vi "Intellirupter_main_WVM.vi"() -> ()   [LabVIEW 2016]
uses:
  <vilib>/Platform/TimedLoop/XDataNode/timing_clust.ctl
  <vilib>/Platform/TimedLoop/XDataNode/nitl_modes.ctl
  <vilib>/Platform/TimedLoop/XDataNode/wakeup.ctl
  <vilib>/FPGAPlugInAG/cRIO-9039 (Sync)/niLvFpga_Open_cRIO-9039 (Sync).vi
  <vilib>/rvi/interface/common/dynamic/niFpgaDynamicAddResources.vi
  <vilib>/Utility/error.llb/Error Cluster From Error Code.vi
  <vilib>/rvi/errors/niLvFpgaAdjustHostInterfaceError.vi
  <vilib>/FPGAPlugInAG/Dynamic/niLvFpga_Close_Dynamic.vi
  <vilib>/rvi/interface/nirviOpenFPGA/nirviOpenFPGA.xnode
  FPGA Bitfiles/IntelliRupter_calibrated.lvbitx
  <vilib>/rvi/interface/nirviReadWriteControl/nirviReadWriteControl.xnode
  <vilib>/Platform/TimedLoop/XDataNode/XDataNode.xnode
  <vilib>/rvi/interface/nirviCloseFPGA/nirviCloseFPGA.xnode
  <vilib>/rvi/interface/Simulation/niFpgaSimulationCallBeginRW.vi
  NiFpgaLv.dll
  <vilib>/Platform/TimedLoop/XDataNode/XDNodeRunTimeDep.lvlib
panel:
  out "basic calc interval":u16=2028
  out "half cycle (samples)":i32=96
  out "Waveform Chart 2":dbl(graph)=58.831625507750715
  in  "I offset R2":dbl=-0.005
  in  "I offset R7":dbl=-0.04
  in  "I offset R3":dbl=-0.12
  out "R8 Transfer":bool
  out "R7 Transfer":bool
  out "R5 Transfer":bool
  out "R4 Transfer":bool
  out "R2 Transfer":bool
  in  "I offset R8":dbl=0.091
  in  "I offset R4":dbl
  in  "I offset R6":dbl=0.092
  in  "I offset R5":dbl=0.035
  in  "I offset R1":dbl=-0.14
  in  "R8 Blocking in":bool
  in  "R7 Blocking in":bool
  in  "R6 Blocking in":bool
  in  "R5 Blocking in":bool
  in  "R4 Blocking in":bool
  in  "R3 Blocking in":bool
  in  "R2 Blocking in":bool
  in  "R1 Blocking in":bool
  out "R1 Blocking out":bool[](array[boolean])
  out "R2 Blocking out":bool[](array[boolean])
  out "R3 Blocking out":bool[](array[boolean])
  out "R4 Blocking out":bool[](array[boolean])
  out "R5 Blocking out":bool[](array[boolean])
  out "R6 Blocking out":bool[](array[boolean])
  out "R8 Blocking out":bool[](array[boolean])
  out "R7 Blocking out":bool[](array[boolean])
  out "Relay7 Reclose":bool=TRUE
  out "Relay7 Trip":bool
  out "Relay8 Reclose":bool=TRUE
  out "Relay8 Trip":bool
  out "Relay6 Reclose":bool=TRUE
  out "Relay6 Trip":bool
  out "Relay5 Reclose":bool=TRUE
  out "Relay5 Trip":bool
  out "Relay4 Reclose":bool=TRUE
  out "Relay4 Trip":bool
  out "Relay3 Reclose":bool=TRUE
  out "Relay3 Trip":bool
  out "Relay2 Reclose":bool=TRUE
  out "Relay2 Trip":bool
  out "Relay1 Reclose":bool=TRUE
  out "Relay1 Trip":bool
  in  "Manual Relay Control":bool
  in  "Reset Relay":bool
  out "Loop time":u32=60
  in  "Recloser Settings":T1={"Magnitude Minimum"=0.1, "Magnitude difference level"=0.1, "Frequency difference level"=0.5, "Phase difference level"=10.0}
  out "MGCC_to_relay":bool[](array[boolean])=[TRUE, TRUE, FALSE, TRUE, TRUE, TRUE, TRUE, TRUE]
  in  "Count(ticks)":u32=10000
  in  "RMS minimum\nvalues":cluster{"VRMS values":dbl, "IRMS values":dbl}={"VRMS values"=0.1, "IRMS values"=0.1}
  out "error out":errorcluster
  out "Relay_toMGCC":bool[](array[boolean])=[TRUE, TRUE, FALSE, TRUE, TRUE, TRUE, TRUE, TRUE]
  in  "Reclose Relay8?":bool=TRUE
  out "R8 Data for\ncommunication":dbl[](array[numeric])=[1.0, 0.9862955093401103, 0.9867214322763603, 58.77451863285861, 58.803693074154864, -0.7941289762119178, 0.09008148312568665, 0.0005073295324109495, 0.0, 0.0]
  in  "Reclose Relay7?":bool=TRUE
  out "R7 Data for\ncommunication":dbl[](array[numeric])=[1.0, 0.9866141364364692, 0.9877614986081782, 58.78358722132554, 58.78069274736454, -1.3449540750541662, 0.08266890794038773, 0.0049254209734499454, 0.0, 0.0]
  in  "Reclose Relay6?":bool=TRUE
  out "R6 Data for\ncommunication":dbl[](array[numeric])=[1.0, 0.9875353501134793, 0.9865248048931855, 58.785757996057974, 58.787154979347115, -1.8287701023872671, 0.08318708091974258, 0.007122902199625969, 0.0, 0.0]
  in  "Reclose Relay5?":bool=TRUE
  out "R5 Data for\ncommunication":dbl[](array[numeric])=[1.0, 0.9886971641324518, 0.9869546019014549, 58.82457095733067, 58.82031783160583, -1.940448004694133, 0.2878004312515259, 0.005543795879930258, 0.0, 0.0]
  in  "Reclose Relay4?":bool=TRUE
  out "R4 Data for\ncommunication":dbl[](array[numeric])=[1.0, 0.9905203551104792, 0.9879386593373192, 58.82435803722625, 58.82419110288083, 1.1327042471490738, 0.28807735443115234, 0.028975406661629677, 0.0, 0.0]
  in  "Reclose Relay3?":bool
  out "R3 Data for\ncommunication":dbl[](array[numeric])=[0.0, 0.9908674808017178, 0.002941768314579481, 81.08898160573632, 58.80421372524394, 60.0, -0.0007620751857757568, -9.880386642180383e-06, 0.0, 0.0]
  in  "Reclose Relay2?":bool=TRUE
  out "R2 Data for\ncommunication":dbl[](array[numeric])=[1.0, 0.9909485571563869, 0.9904603427539119, 58.813573202375395, 58.79227178425196, 0.9332438342282595, 0.38369542360305786, 0.024205466732382774, 0.0, -0.021301418123435667]
  out "R1 Data for\ncommunication":dbl[](array[numeric])=[1.0, 0.9931811773356323, 0.9935607508678418, 58.852139713340016, 58.831625507750715, 0.5044340052335675, 0.4828683137893677, 0.0162374097853899, 0.0, -0.020514205589300616]
  in  "Relay8":bool=TRUE
  in  "Relay7":bool=TRUE
  in  "Relay6":bool=TRUE
  in  "Relay5":bool=TRUE
  in  "Relay4":bool=TRUE
  in  "Relay3":bool
  in  "Relay2":bool=TRUE
  in  "Reclose Relay1?":bool=TRUE
  in  "stop":bool
  in  "Relay1":bool=TRUE
  # "status\nmag_left\nmag_right\nfreq_left\nfreq_right\nang_diff\nact_power\nrea_power\n0\n0"
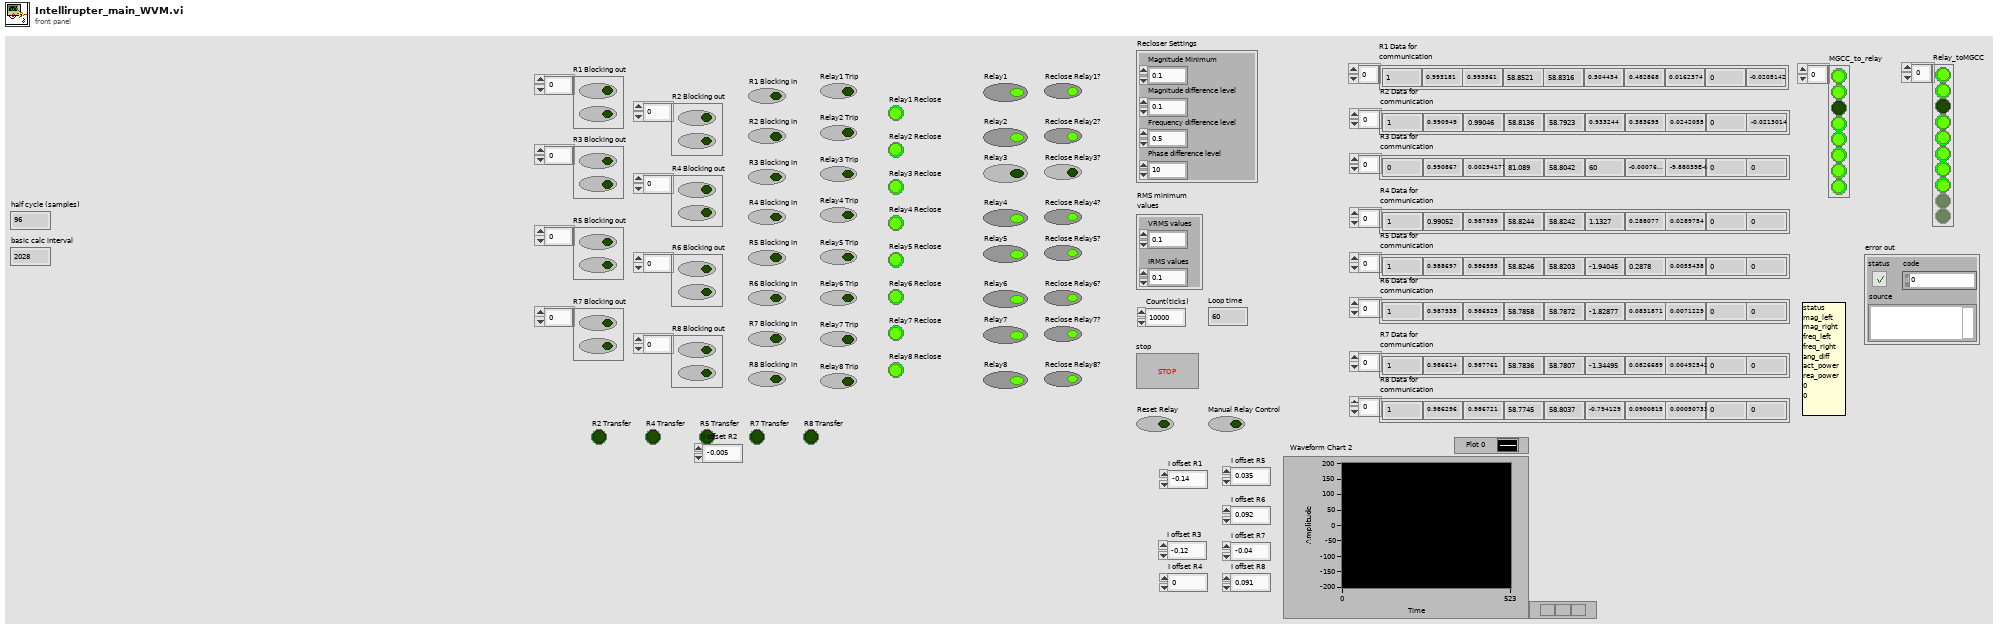
[diagram p1: front panel]
types:
  T1 = cluster{"Magnitude Minimum":dbl, "Magnitude difference level":dbl, "Frequency difference level":dbl, "Phase difference level":dbl}
  T2 = typedef "XDNodeRunTimeDep.lvlib/timing_clust.ctl" = cluster{"Expected End [f-1]":u64, "Actual End [f-1]":u64, "Finished Late? [f-1]":bool, "Expected End [i-1]":u64, "Actual End [i-1]":u64, "Finished Late? [i-1]":bool, "Expected Start [i]":u64, "Actual Start [i]":u64, "Expected Start [f]":u64, "Actual Start [f]":u64, "Source Name":string, "Structure Name":string, "Period":i64, "Deadline":i64, "Offset":i64, "Start":i64, "Priority":i32, "Timeout":i32, "Mode":T3, "Wakeup Reason":T4, "Error":errorcluster, "Source Type":string, "Secondary Source Type":string, "Global End Time":u64, "Global Start Time":u64, "Frame Duration":u64, "Iteration Duration":u64, "Assigned CPU":i32, "I/O Scan Engine Mode":u32}
  T3 = typedef "XDNodeRunTimeDep.lvlib/nitl_modes.ctl" = enum32{"No Change", "Process missed periods, maintain original phase", "Discard missed periods, maintain original phase", "Process missed periods, ignore original phase", "Discard missed periods, ignore original phase"}
  T4 = typedef "XDNodeRunTimeDep.lvlib/wakeup.ctl" = enum32{"Normal", "Aborted", "Asynchronous wakeup", "Timing source error", "Timed loop error", "Timeout"}
  T5 = enum16{"Grid-connected", "BESS only", "PV + BESS"}
  T6 = cluster{"UV Reset level":dbl, "Undervoltage \npick-up level":dbl, "OC Reset level":dbl, "Overcurrent\npick-up level":dbl, "time delay settings":cluster{"Definite operate time [ms]":u32, "Inverse Operating Time [ms]":u32, "reset time [ms]":u32, "operate time compensation [ms]":u32}}
  T7 = cluster{fxp<+/-,53,11>[], fxp<+/-,53,11>[], fxp<+/-,53,11>[], fxp<+/-,53,11>[], fxp<+/-,53,11>[], fxp<+/-,53,11>[], fxp<+/-,53,11>[], fxp<+/-,53,11>[], fxp<+/-,53,11>[]}
  T8 = typedef "NI_EP_Protection_FPGA.lvlib/fpga_Timer Feedback Var.ctl" = cluster{"time elapsed":u32, "start time of trip counting":u32, "start time of reseting":u32}
  T9 = typedef "NI_EP_Protection_FPGA.lvlib/fpga_State.ctl" = enum16{"Idle", "Trip Counting", "Tripped", "Reset Counting"}
  T10 = cluster{"Direction":enum16{"forward", "backward", "N/D"}, "Boolean":bool, "timing values out":T8, "status out":T9, "trip signal out":bool, "State Out":enum16{"Idle", "Wait for Trip", "PulseClosing", "Locked"}, "Pulse Index Out":i32, "start time of reseting":u32}
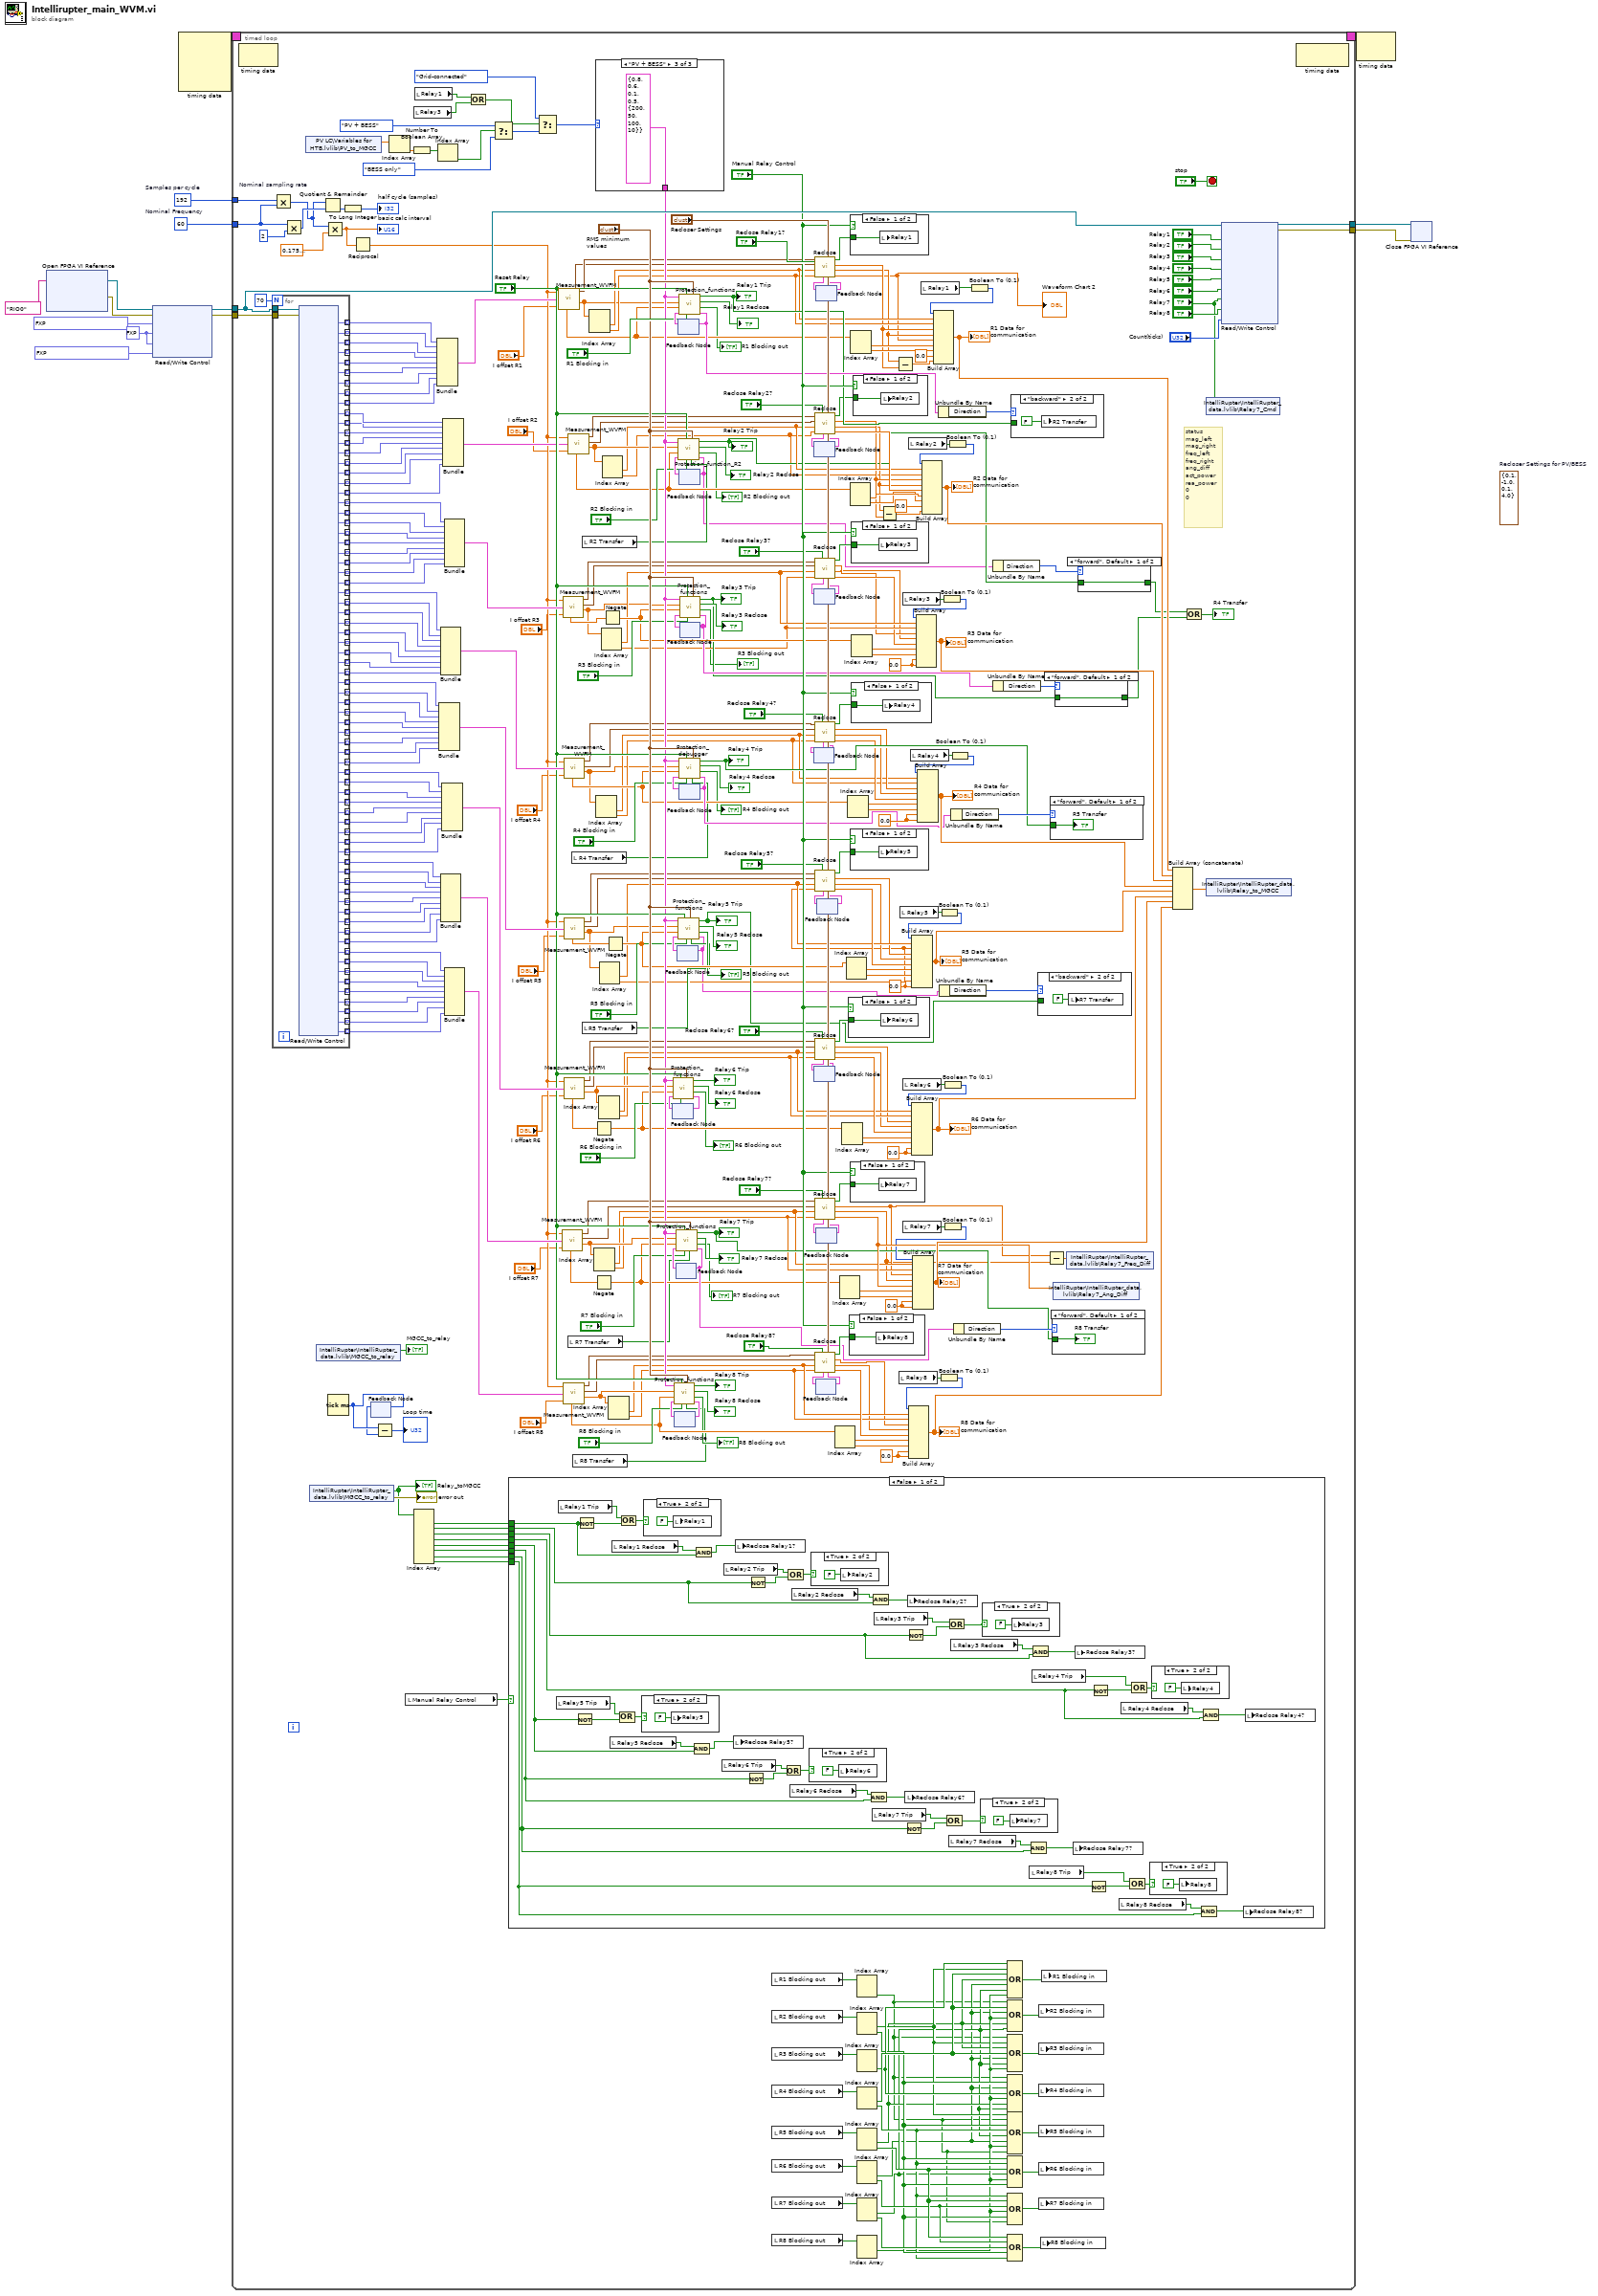
[diagram p0: block diagram]
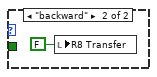
[diagram p2: hidden frame]
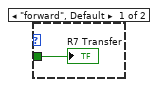
[diagram p3: hidden frame]
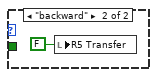
[diagram p4: hidden frame]
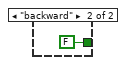
[diagram p5: hidden frame]
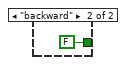
[diagram p6: hidden frame]
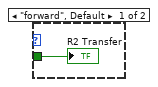
[diagram p7: hidden frame]
diagram:
  w2 = 192  # Samples per cycle
  w1 = 60  # Nominal Frequency
  (unwired) T1 {"Magnitude Minimum"=0.1, "Magnitude difference level"=-1.0, "Frequency difference level"=0.1, "Phase difference level"=4.0}  # Recloser Settings for PV/BESS
  w6 = fxp<+/-,52,10> 0.0 ("I offset")
  n1 = xnode "Open FPGA VI Reference"("resource name"=tag "RIO0") -> ("FPGA VI Reference Out"=w5:refnum<k20>, "error out"=w10:errorcluster)  [unwired: 1 in]
  n2 = xnode "Read/Write Control"("FPGA VI Reference In"=w5, "error in"=w10, "I scale factor"=fxp<+/-,26,5> 0.4850001335144043, "I offset"=w6, "V offset"=w6, "V scale factor"=fxp<+/-,26,5> 0.40000009536743164) -> ("FPGA VI Reference Out"=w11:refnum<k20>, "error out"=w9:errorcluster)
  n3 = node-c288() -> (w4:T2)  [unwired: 4 in]
  n4 = timed-loop {
    tunnel: w11 -> [w407]
    tunnel: [w409] -> w13
    tunnel: [w408] -> w12
    tunnel: w9 -> [w406]
    timing: w4 -> [_]
    timing-out: [_] -> w3
    tunnel: w2 -> [w86]
    tunnel: w1 -> [w85]
    stop <- "stop" stop-if-true
    w243 = 0.0 ("element")
    w244 = 0.0 ("element")
    w256 = 0.0 ("element")
    w127 = 0.0 ("element")
    w268 = 0.0 ("element")
    w269 = 0.0 ("element")
    # "status\nmag_left\nmag_right\nfreq_left\nfreq_right\nang_diff\nact_power\nrea_power\n0\n0"
    n5 = node-c288() -> ()  [unwired: 1 in, 1 out]
    n6 = for {
      N: 70 -> [_]
      tunnel: w407 -> [w484]
      tunnel: w406 -> [w483]
      tunnel: [w482] -> w405 mode=indexing
      tunnel: [w481] -> w404 mode=indexing
      tunnel: [w480] -> w403 mode=indexing
      tunnel: [w479] -> w402 mode=indexing
      tunnel: [w478] -> w401 mode=indexing
      tunnel: [w477] -> w400 mode=indexing
      tunnel: [w476] -> w399 mode=indexing
      tunnel: [w475] -> w398 mode=indexing
      tunnel: [w474] -> w386 mode=indexing
      tunnel: [w473] -> w385 mode=indexing
      tunnel: [w472] -> w384 mode=indexing
      tunnel: [w471] -> w383 mode=indexing
      tunnel: [w470] -> w382 mode=indexing
      tunnel: [w469] -> w381 mode=indexing
      tunnel: [w468] -> w380 mode=indexing
      tunnel: [w467] -> w379 mode=indexing
      tunnel: [w466] -> w378 mode=indexing
      tunnel: [w465] -> w377 mode=indexing
      tunnel: [w464] -> w376 mode=indexing
      tunnel: [w463] -> w375 mode=indexing
      tunnel: [w462] -> w374 mode=indexing
      tunnel: [w461] -> w373 mode=indexing
      tunnel: [w460] -> w372 mode=indexing
      tunnel: [w459] -> w371 mode=indexing
      tunnel: [w458] -> w370 mode=indexing
      tunnel: [w457] -> w369 mode=indexing
      tunnel: [w456] -> w368 mode=indexing
      tunnel: [w455] -> w367 mode=indexing
      tunnel: [w454] -> w366 mode=indexing
      tunnel: [w453] -> w365 mode=indexing
      tunnel: [w452] -> w364 mode=indexing
      tunnel: [w451] -> w363 mode=indexing
      tunnel: [w450] -> w362 mode=indexing
      tunnel: [w449] -> w361 mode=indexing
      tunnel: [w448] -> w360 mode=indexing
      tunnel: [w447] -> w359 mode=indexing
      tunnel: [w446] -> w358 mode=indexing
      tunnel: [w445] -> w357 mode=indexing
      tunnel: [w444] -> w356 mode=indexing
      tunnel: [w443] -> w355 mode=indexing
      tunnel: [w442] -> w354 mode=indexing
      tunnel: [w441] -> w353 mode=indexing
      tunnel: [w440] -> w352 mode=indexing
      tunnel: [w439] -> w351 mode=indexing
      tunnel: [w438] -> w350 mode=indexing
      tunnel: [w437] -> w349 mode=indexing
      tunnel: [w436] -> w348 mode=indexing
      tunnel: [w435] -> w347 mode=indexing
      tunnel: [w434] -> w346 mode=indexing
      tunnel: [w433] -> w345 mode=indexing
      tunnel: [w432] -> w344 mode=indexing
      tunnel: [w431] -> w343 mode=indexing
      tunnel: [w430] -> w342 mode=indexing
      tunnel: [w429] -> w341 mode=indexing
      tunnel: [w428] -> w340 mode=indexing
      tunnel: [w427] -> w339 mode=indexing
      tunnel: [w426] -> w338 mode=indexing
      tunnel: [w425] -> w337 mode=indexing
      tunnel: [w424] -> w336 mode=indexing
      tunnel: [w423] -> w335 mode=indexing
      tunnel: [w422] -> w334 mode=indexing
      tunnel: [w421] -> w333 mode=indexing
      tunnel: [w420] -> w280 mode=indexing
      tunnel: [w419] -> w184 mode=indexing
      tunnel: [w418] -> w183 mode=indexing
      tunnel: [w417] -> w182 mode=indexing
      tunnel: [w416] -> w181 mode=indexing
      tunnel: [w415] -> w180 mode=indexing
      tunnel: [w414] -> w179 mode=indexing
      tunnel: [w413] -> w178 mode=indexing
      tunnel: [w412] -> w177 mode=indexing
      tunnel: [w411] -> w176 mode=indexing
      n7 = xnode "Read/Write Control"("FPGA VI Reference In"=w484, "error in"=w483) -> ("V1L AB"=w420:fxp<+/-,53,11>, "V1L BC"=w482:fxp<+/-,53,11>, "V1L CA"=w481:fxp<+/-,53,11>, "V1R AB"=w480:fxp<+/-,53,11>, "V1R BC"=w479:fxp<+/-,53,11>, "V1R CA"=w478:fxp<+/-,53,11>, "I1 A"=w477:fxp<+/-,53,11>, "I1 B"=w476:fxp<+/-,53,11>, "I1 C"=w475:fxp<+/-,53,11>, "V2L AB"=w419:fxp<+/-,53,11>, "V2L BC"=w418:fxp<+/-,53,11>, "V2L CA"=w417:fxp<+/-,53,11>, "V2R AB"=w416:fxp<+/-,53,11>, "V2R BC"=w415:fxp<+/-,53,11>, "V2R CA"=w414:fxp<+/-,53,11>, "I2 A"=w413:fxp<+/-,53,11>, "I2 B"=w412:fxp<+/-,53,11>, "I2 C"=w411:fxp<+/-,53,11>, "V3L AB"=w474:fxp<+/-,53,11>, "V3L BC"=w473:fxp<+/-,53,11>, "V3L CA"=w472:fxp<+/-,53,11>, "V3R AB"=w471:fxp<+/-,53,11>, "V3R BC"=w470:fxp<+/-,53,11>, "V3R CA"=w469:fxp<+/-,53,11>, "I3 A"=w468:fxp<+/-,53,11>, "I3 B"=w467:fxp<+/-,53,11>, "I3 C"=w466:fxp<+/-,53,11>, "V4L AB"=w465:fxp<+/-,53,11>, "V4L BC"=w464:fxp<+/-,53,11>, "V4L CA"=w463:fxp<+/-,53,11>, "V4R AB"=w462:fxp<+/-,53,11>, "V4R BC"=w461:fxp<+/-,53,11>, "V4R CA"=w460:fxp<+/-,53,11>, "I4 A"=w459:fxp<+/-,53,11>, "I4 B"=w458:fxp<+/-,53,11>, "I4 C"=w457:fxp<+/-,53,11>, "V5L AB"=w456:fxp<+/-,53,11>, "V5L BC"=w455:fxp<+/-,53,11>, "V5L CA"=w454:fxp<+/-,53,11>, "V5R AB"=w453:fxp<+/-,53,11>, "V5R BC"=w452:fxp<+/-,53,11>, "V5R CA"=w451:fxp<+/-,53,11>, "I5 A"=w450:fxp<+/-,53,11>, "I5 B"=w449:fxp<+/-,53,11>, "I5 C"=w448:fxp<+/-,53,11>, "V6L AB"=w447:fxp<+/-,53,11>, "V6L BC"=w446:fxp<+/-,53,11>, "V6L CA"=w445:fxp<+/-,53,11>, "V6R AB"=w444:fxp<+/-,53,11>, "V6R BC"=w443:fxp<+/-,53,11>, "V6R CA"=w442:fxp<+/-,53,11>, "I6 A"=w441:fxp<+/-,53,11>, "I6 B"=w440:fxp<+/-,53,11>, "I6 C"=w439:fxp<+/-,53,11>, "V7L AB"=w438:fxp<+/-,53,11>, "V7L BC"=w437:fxp<+/-,53,11>, "V7L CA"=w436:fxp<+/-,53,11>, "V7R AB"=w435:fxp<+/-,53,11>, "V7R BC"=w434:fxp<+/-,53,11>, "V7R CA"=w433:fxp<+/-,53,11>, "I7 A"=w432:fxp<+/-,53,11>, "I7 B"=w431:fxp<+/-,53,11>, "I7 C"=w430:fxp<+/-,53,11>, "V8L AB"=w429:fxp<+/-,53,11>, "V8L BC"=w428:fxp<+/-,53,11>, "V8L CA"=w427:fxp<+/-,53,11>, "V8R AB"=w426:fxp<+/-,53,11>, "V8R BC"=w425:fxp<+/-,53,11>, "V8R CA"=w424:fxp<+/-,53,11>, "I8 A"=w423:fxp<+/-,53,11>, "I8 B"=w422:fxp<+/-,53,11>, "I8 C"=w421:fxp<+/-,53,11>)  [unwired: 2 out]
    }
    n8 = Multiply "Nominal sampling rate"(x=w86, y=w85) -> (x*y=w88:i32)
    n9 = Multiply(x=w85, y=2) -> (x*y=w92:i32)
    n10 = shared-variable "PV LC\\Variables for HTB.lvlib\\PV_to_MGCC"() -> (w74:dbl[])  [unwired: 1 in, 1 out]
    n11 = shared-variable "IntelliRupter\\IntelliRupter_data.lvlib\\MGCC_to_relay"() -> (w320:bool[], error out=→"error out":errorcluster)  [unwired: 1 in]
    "Relay_toMGCC" <- w320
    n12 = shared-variable "IntelliRupter\\IntelliRupter_data.lvlib\\MGCC_to_relay"() -> (→"MGCC_to_relay":bool[])  [unwired: 1 in, 1 out]
    n13 = Quotient & Remainder(x=w88, y=w92) -> (floor(x/y)=w90:i32)  [unwired: 1 out]
    n14 = Multiply(x=w88, y=sgl 0.176 ("y 2")) -> (x*y=w87:sgl)
    "basic calc interval" <- w87
    n15 = Tick Count (ms)() -> (millisecond timer value=w311:u32)
    n16 = To Long Integer(number=w90) -> (32bit integer=→"half cycle (samples)":i32)
    n17 = Reciprocal(x=w87) -> (1/x=w84:sgl)
    n18 = feedback #1() -> (w310:u32)  [unwired: 1 in]
    n19 = feedback-in #1(w311) -> ()
    n20 = Subtract(x=w311, y=w310) -> (x-y=→"Loop time":u32)
    n21 = Index Array(array=w74) -> (element=w317:dbl)  [unwired: 1 in]
    n22 = local read "Manual Relay Control"() -> (w290:bool)
    n23 = Number To Boolean Array(number=w317) -> (Boolean array=w316:bool[])
    n24 = local read "Relay3"() -> (w22:bool)
    n25 = Index Array(array=w320) -> (element #1=w298:bool, element #2=w297:bool, element #3=w296:bool, element #4=w295:bool, element #5=w294:bool, element #6=w293:bool, element #7=w292:bool, element #8=w291:bool)  [unwired: 8 in]
    n26 = local read "Relay1"() -> (w23:bool)
    n27 = Bundle(w280, w405, w404, w403, w402, w401, w400, w399, w398) -> (w170:T7)  [unwired: 1 in]
    n28 = Index Array(array=w316) -> (element=w315:bool)  [unwired: 1 in]
    n29 = Bundle(w368, w367, w366, w365, w364, w363, w362, w361, w360) -> (w306:T7)  [unwired: 1 in]
    n30 = Bundle(w377, w376, w375, w374, w373, w372, w371, w370, w369) -> (w307:T7)  [unwired: 1 in]
    n31 = Bundle(w350, w349, w348, w347, w346, w345, w344, w343, w342) -> (w304:T7)  [unwired: 1 in]
    n32 = Bundle(w359, w358, w357, w356, w355, w354, w353, w352, w351) -> (w305:T7)  [unwired: 1 in]
    n33 = Bundle(w184, w183, w182, w181, w180, w179, w178, w177, w176) -> (w175:T7)  [unwired: 1 in]
    n34 = Bundle(w386, w385, w384, w383, w382, w381, w380, w379, w378) -> (w308:T7)  [unwired: 1 in]
    n35 = Bundle(w341, w340, w339, w338, w337, w336, w335, w334, w333) -> (w303:T7)  [unwired: 1 in]
    n36 = Or(x=w23, y=w22) -> (x .or. y?=w21:bool)
    n37 = Select(t=T5."PV + BESS", s=w315, f=T5."BESS only") -> (s? t:f=w24:T5)
    n38 = case shown="False" w290 {
      tunnel: w298 -> [w539 _]
      tunnel: w297 -> [w537 _]
      tunnel: w296 -> [w533 _]
      tunnel: w295 -> [w530 _]
      tunnel: w294 -> [w509 _]
      tunnel: w293 -> [w508 _]
      tunnel: w292 -> [w507 _]
      tunnel: w291 -> [w506 _]
      frame False {
        n39 = local read "Relay5 Trip"() -> (w510:bool)
        n40 = local read "Relay1 Trip"() -> (w553:bool)
        n41 = Not(x=w509) -> (.not. x?=w512:bool)
        n42 = Not(x=w539) -> (.not. x?=w551:bool)
        n43 = local read "Relay5 Reclose"() -> (w523:bool)
        n44 = local read "Relay1 Reclose"() -> (w540:bool)
        n45 = Or(x=w553, y=w551) -> (x .or. y?=w552:bool)
        n46 = Compound Arithmetic op=OR(w510, w512) -> (w511:bool)
        n47 = case shown="True" w511 {
          frame False {
          }
          frame True {
            n48 = local write "Relay5"(FALSE ("Relay8")) -> ()
          }
        }
        n49 = case shown="True" w552 {
          frame False {
          }
          frame True {
            n50 = local write "Relay1"(FALSE ("Relay8")) -> ()
          }
        }
        n51 = And(x=w540, y=w539) -> (x .and. y?=w541:bool)
        n52 = Compound Arithmetic op=AND(w523, w509) -> (w522:bool)
        n53 = local read "Relay6 Trip"() -> (w519:bool)
        n54 = local read "Relay2 Trip"() -> (w544:bool)
        n55 = local write "Reclose Relay5?"(w522) -> ()
        n56 = local write "Reclose Relay1?"(w541) -> ()
        n57 = Not(x=w508) -> (.not. x?=w513:bool)
        n58 = Not(x=w537) -> (.not. x?=w550:bool)
        n59 = Or(x=w519, y=w513) -> (x .or. y?=w514:bool)
        n60 = Compound Arithmetic op=OR(w544, w550) -> (w549:bool)
        n61 = local read "Relay6 Reclose"() -> (w525:bool)
        n62 = local read "Relay2 Reclose"() -> (w536:bool)
        n63 = case shown="True" w514 {
          frame False {
          }
          frame True {
            n64 = local write "Relay6"(FALSE ("Relay8")) -> ()
          }
        }
        n65 = case shown="True" w549 {
          frame False {
          }
          frame True {
            n66 = local write "Relay2"(FALSE ("Relay8")) -> ()
          }
        }
        n67 = And(x=w525, y=w508) -> (x .and. y?=w524:bool)
        n68 = local read "Relay7 Trip"() -> (w520:bool)
        n69 = Compound Arithmetic op=AND(w536, w537) -> (w538:bool)
        n70 = local read "Relay3 Trip"() -> (w543:bool)
        n71 = Not(x=w507) -> (.not. x?=w516:bool)
        n72 = local write "Reclose Relay6?"(w524) -> ()
        n73 = Not(x=w533) -> (.not. x?=w547:bool)
        n74 = local write "Reclose Relay2?"(w538) -> ()
        n75 = Or(x=w543, y=w547) -> (x .or. y?=w548:bool)
        n76 = Compound Arithmetic op=OR(w520, w516) -> (w515:bool)
        n77 = local read "Relay7 Reclose"() -> (w527:bool)
        n78 = local read "Relay3 Reclose"() -> (w534:bool)
        n79 = case shown="True" w515 {
          frame False {
          }
          frame True {
            n80 = local write "Relay7"(FALSE ("Relay8")) -> ()
          }
        }
        n81 = case shown="True" w548 {
          frame False {
          }
          frame True {
            n82 = local write "Relay3"(FALSE ("Relay8")) -> ()
          }
        }
        n83 = local read "Relay8 Trip"() -> (w521:bool)
        n84 = And(x=w534, y=w533) -> (x .and. y?=w535:bool)
        n85 = Compound Arithmetic op=AND(w527, w507) -> (w526:bool)
        n86 = local read "Relay4 Trip"() -> (w542:bool)
        n87 = local write "Reclose Relay7?"(w526) -> ()
        n88 = local write "Reclose Relay3?"(w535) -> ()
        n89 = Not(x=w506) -> (.not. x?=w517:bool)
        n90 = Not(x=w530) -> (.not. x?=w546:bool)
        n91 = local read "Relay8 Reclose"() -> (w528:bool)
        n92 = local read "Relay4 Reclose"() -> (w532:bool)
        n93 = Compound Arithmetic op=OR(w521, w517) -> (w518:bool)
        n94 = Compound Arithmetic op=OR(w542, w546) -> (w545:bool)
        n95 = case shown="True" w518 {
          frame False {
          }
          frame True {
            n96 = local write "Relay8"(FALSE ("Relay8")) -> ()
          }
        }
        n97 = case shown="True" w545 {
          frame False {
          }
          frame True {
            n98 = local write "Relay4"(FALSE ("Relay8")) -> ()
          }
        }
        n99 = Compound Arithmetic op=AND(w528, w506) -> (w529:bool)
        n100 = Compound Arithmetic op=AND(w532, w530) -> (w531:bool)
        n101 = local write "Reclose Relay8?"(w529) -> ()
        n102 = local write "Reclose Relay4?"(w531) -> ()
      }
      frame True {
      }
    }
    n103 = Select(t=T5."Grid-connected", s=w21, f=w24) -> (s? t:f=w25:T5)
    n104 = call "Measurement_WVFM.vi"("dt"=w84, "Input cluster"=w170, "Ioffset"="I offset R1") -> ("Total power values"=w156:dbl[], "VL array"=w166:waveform(sgl)[], "VR array"=w165:waveform(sgl)[], "RMS values"=w160:dbl[])  [unwired: 1 in, 1 out]
    n105 = call "Measurement_WVFM.vi"("dt"=w84, "Input cluster"=w304, "Ioffset"="I offset R7") -> ("Total power values"=w111:dbl[], "VL array"=w110:waveform(sgl)[], "VR array"=w109:waveform(sgl)[], "RMS values"=w108:dbl[])  [unwired: 1 in, 1 out]
    n106 = call "Measurement_WVFM.vi"("dt"=w84, "Input cluster"=w308, "Ioffset"="I offset R3") -> ("Total power values"=w144:dbl[], "VL array"=w146:waveform(sgl)[], "VR array"=w145:waveform(sgl)[], "RMS values"=w122:dbl[])  [unwired: 1 in, 1 out]
    n107 = call "Measurement_WVFM.vi"("dt"=w84, "Input cluster"=w303, "Ioffset"="I offset R8") -> ("Total power values"=w103:dbl[], "VL array"=w102:waveform(sgl)[], "VR array"=w101:waveform(sgl)[], "RMS values"=w100:dbl[])  [unwired: 1 in, 1 out]
    n108 = call "Measurement_WVFM.vi"("dt"=w84, "Input cluster"=w307, "Ioffset"="I offset R4") -> ("Total power values"=w140:dbl[], "VL array"=w136:waveform(sgl)[], "VR array"=w137:waveform(sgl)[], "RMS values"=w123:dbl[])  [unwired: 1 in, 1 out]
    n109 = call "Measurement_WVFM.vi"("dt"=w84, "Input cluster"=w306, "Ioffset"="I offset R5") -> ("Total power values"=w129:dbl[], "VL array"=w131:waveform(sgl)[], "VR array"=w130:waveform(sgl)[], "RMS values"=w124:dbl[])  [unwired: 1 in, 1 out]
    n110 = call "Measurement_WVFM.vi"("dt"=w84, "Input cluster"=w305, "Ioffset"="I offset R6") -> ("Total power values"=w121:dbl[], "VL array"=w119:waveform(sgl)[], "VR array"=w118:waveform(sgl)[], "RMS values"=w120:dbl[])  [unwired: 1 in, 1 out]
    n111 = call "Measurement_WVFM.vi"("dt"=w84, "Input cluster"=w175, "Ioffset"="I offset R2") -> ("Total power values"=w155:dbl[], "VL array"=w158:waveform(sgl)[], "VR array"=w157:waveform(sgl)[], "RMS values"=w154:dbl[])  [unwired: 1 in, 1 out]
    n112 = local read "R7 Transfer"() -> (w64:bool)
    n113 = local read "R4 Transfer"() -> (w62:bool)
    n114 = local read "R8 Transfer"() -> (w65:bool)
    n115 = local read "R5 Transfer"() -> (w63:bool)
    n116 = local read "R2 Transfer"() -> (w61:bool)
    n117 = Index Array(array=w160) -> (element #1=w164:dbl, element #2=w163:dbl)  [unwired: 2 in]
    n118 = Negate(x=w121) -> (-x=w186:dbl[])
    n119 = Index Array(array=w108) -> (element #1=w107:dbl, element #2=w106:dbl)  [unwired: 2 in]
    n120 = Negate(x=w111) -> (-x=w185:dbl[])
    n121 = case shown="\"PV + BESS\"" w25 {
      tunnel: [T6 {"UV Reset level"=0.9, "Undervoltage \npick-up level"=0.8, "OC Reset level"=0.1, "Overcurrent\npick-up level"=0.5, "time delay settings"={"Definite operate time [ms]"=120, "Inverse Operating Time [ms]"=100, "reset time [ms]"=100, "operate time compensation [ms]"=10}} ("Protection settings") T6 {"UV Reset level"=0.7, "Undervoltage \npick-up level"=0.5, "OC Reset level"=0.1, "Overcurrent\npick-up level"=0.17, "time delay settings"={"Definite operate time [ms]"=400, "Inverse Operating Time [ms]"=45, "reset time [ms]"=100, "operate time compensation [ms]"=10}} ("Protection settings") T6 {"UV Reset level"=0.8, "Undervoltage \npick-up level"=0.6, "OC Reset level"=0.1, "Overcurrent\npick-up level"=0.5, "time delay settings"={"Definite operate time [ms]"=200, "Inverse Operating Time [ms]"=50, "reset time [ms]"=100, "operate time compensation [ms]"=10}} ("Protection settings")] -> w285
      frame "Grid-connected", Default {
      }
      frame "BESS only" {
      }
      frame "PV + BESS" {
      }
    }
    n122 = Index Array(array=w123) -> (element #1=w135:dbl, element #2=w134:dbl)  [unwired: 2 in]
    n123 = Index Array(array=w120) -> (element #1=w115:dbl, element #2=w114:dbl)  [unwired: 2 in]
    n124 = Index Array(array=w124) -> (element #1=w128:dbl, element #2=w57:dbl)  [unwired: 2 in]
    n125 = Index Array(array=w122) -> (element #1=w148:dbl, element #2=w147:dbl)  [unwired: 2 in]
    n126 = Index Array(array=w154) -> (element #1=w153:dbl, element #2=w58:dbl)  [unwired: 2 in]
    n127 = Negate(x=w144) -> (-x=w199:dbl[])
    n128 = Negate(x=w129) -> (-x=w201:dbl[])
    n129 = Index Array(array=w100) -> (element #1=w97:dbl, element #2=w96:dbl)  [unwired: 2 in]
    n130 = feedback #2() -> (w229:T10)  [unwired: 1 in]
    n131 = call "Protection_functions.vi"("RMS minimum\nvalues"="RMS minimum\nvalues", "Blocking in"="R6 Blocking in", "Reset Relay"="Reset Relay", "input cluster"=w229, "Total power values"=w186, "RMS values"=w120, "Protection settings"=w285) -> ("output cluster"=w230:T10, "Blocking out"=→"R6 Blocking out":bool[], "Reclose"=→"Relay6 Reclose":bool, "trip signal"=→"Relay6 Trip":bool)  [unwired: 1 in]
    n132 = feedback-in #2(w230) -> ()
    n133 = feedback #3() -> (w226:T10)  [unwired: 1 in]
    n134 = call "Protection_functions.vi"("Transfer Trip"=w65, "RMS minimum\nvalues"="RMS minimum\nvalues", "Blocking in"="R8 Blocking in", "Reset Relay"="Reset Relay", "input cluster"=w226, "Total power values"=w103, "RMS values"=w100, "Protection settings"=w285) -> ("output cluster"=w227:T10, "Blocking out"=→"R8 Blocking out":bool[], "Reclose"=→"Relay8 Reclose":bool, "trip signal"=→"Relay8 Trip":bool)
    n135 = feedback-in #3(w227) -> ()
    n136 = feedback #4() -> (w228:T10)  [unwired: 1 in]
    n137 = call "Protection_functions.vi"("Transfer Trip"=w64, "RMS minimum\nvalues"="RMS minimum\nvalues", "Blocking in"="R7 Blocking in", "Reset Relay"="Reset Relay", "input cluster"=w228, "Total power values"=w185, "RMS values"=w108, "Protection settings"=w285) -> ("output cluster"=w189:T10, "Blocking out"=→"R7 Blocking out":bool[], "Reclose"=→"Relay7 Reclose":bool, "trip signal"=w187:bool)
    "Relay7 Trip" <- w187
    n138 = feedback-in #4(w189) -> ()
    n139 = feedback #5() -> (w204:T10)  [unwired: 1 in]
    n140 = feedback #6() -> (w301:T10)  [unwired: 1 in]
    n141 = call "Protection_functions.vi"("Transfer Trip"=w63, "RMS minimum\nvalues"="RMS minimum\nvalues", "Blocking in"="R5 Blocking in", "Reset Relay"="Reset Relay", "input cluster"=w204, "Total power values"=w201, "RMS values"=w124, "Protection settings"=w285) -> ("output cluster"=w55:T10, "Blocking out"=→"R5 Blocking out":bool[], "Reclose"=→"Relay5 Reclose":bool, "trip signal"=w190:bool)
    "Relay5 Trip" <- w190
    n142 = feedback-in #5(w55) -> ()
    n143 = call "Protection_functions.vi"("RMS minimum\nvalues"="RMS minimum\nvalues", "Blocking in"="R1 Blocking in", "Reset Relay"="Reset Relay", "input cluster"=w301, "Total power values"=w156, "RMS values"=w160, "Protection settings"=w285) -> ("output cluster"=w284:T10, "Blocking out"=→"R1 Blocking out":bool[], "Reclose"=→"Relay1 Reclose":bool, "trip signal"=w283:bool)  [unwired: 1 in]
    "Relay1 Trip" <- w283
    n144 = feedback-in #6(w284) -> ()
    n145 = feedback #7() -> (w232:T10)  [unwired: 1 in]
    n146 = call "Protection_function_R2.vi"("Transfer Trip"=w61, "RMS minimum\nvalues"="RMS minimum\nvalues", "Blocking in"="R2 Blocking in", "Reset Relay"="Reset Relay", "input cluster"=w232, "Total power values"=w155, "RMS values"=w154, "Protection settings"=w285) -> ("output cluster"=w56:T10, "Blocking out"=→"R2 Blocking out":bool[], "Reclose"=→"Relay2 Reclose":bool, "trip signal"=w59:bool)
    "Relay2 Trip" <- w59
    n147 = feedback-in #7(w56) -> ()
    n148 = feedback #8() -> (w231:T10)  [unwired: 1 in]
    n149 = call "Protection_debugger.vi"("Transfer Trip"=w62, "RMS minimum\nvalues"="RMS minimum\nvalues", "Blocking in"="R4 Blocking in", "Reset Relay"="Reset Relay", "input cluster"=w231, "Total power values"=w140, "RMS values"=w123, "Protection settings"=w285) -> ("output cluster"=w194:T10, "Blocking out"=→"R4 Blocking out":bool[], "Reclose"=→"Relay4 Reclose":bool, "trip signal"=w192:bool)
    "Relay4 Trip" <- w192
    n150 = feedback-in #8(w194) -> ()
    n151 = feedback #9() -> (w233:T10)  [unwired: 1 in]
    n152 = call "Protection_functions.vi"("RMS minimum\nvalues"="RMS minimum\nvalues", "Blocking in"="R3 Blocking in", "Reset Relay"="Reset Relay", "input cluster"=w233, "Total power values"=w199, "RMS values"=w122, "Protection settings"=w285) -> ("output cluster"=w196:T10, "Blocking out"=→"R3 Blocking out":bool[], "Reclose"=→"Relay3 Reclose":bool, "trip signal"=w195:bool)  [unwired: 1 in]
    "Relay3 Trip" <- w195
    n153 = feedback-in #9(w196) -> ()
    n154 = local read "R1 Blocking out"() -> (w54:bool[])
    n155 = local read "R2 Blocking out"() -> (w53:bool[])
    n156 = local read "R3 Blocking out"() -> (w52:bool[])
    n157 = local read "R4 Blocking out"() -> (w51:bool[])
    n158 = local read "R5 Blocking out"() -> (w50:bool[])
    n159 = local read "R6 Blocking out"() -> (w49:bool[])
    n160 = local read "R7 Blocking out"() -> (w48:bool[])
    n161 = local read "R8 Blocking out"() -> (w47:bool[])
    n162 = feedback #10() -> (w138:cluster{bool, dbl})  [unwired: 1 in]
    n163 = feedback #11() -> (w159:cluster{bool, dbl})  [unwired: 1 in]
    n164 = feedback #12() -> (w149:cluster{bool, dbl})  [unwired: 1 in]
    n165 = feedback #13() -> (w116:cluster{bool, dbl})  [unwired: 1 in]
    n166 = call "Reclose.vi"("Recloser Settings"="Recloser Settings", "Recloser in"=w159, "Reclose?"="Reclose Relay2?", "VR RMS avg"=w58, "VL RMS avg"=w153, "VR array"=w157, "VL array"=w158) -> ("Phase difference"=w171:dbl, "VR Frequency"=w151:dbl, "VL Frequency"=w152:dbl, "Recloser action"=w217:bool, "Recloser out"=w274:cluster{bool, dbl})
    n167 = feedback-in #11(w274) -> ()
    n168 = call "Reclose.vi"("Recloser Settings"="Recloser Settings", "Recloser in"=w149, "Reclose?"="Reclose Relay3?", "VR RMS avg"=w147, "VL RMS avg"=w148, "VR array"=w145, "VL array"=w146) -> ("Phase difference"=w17:dbl, "VR Frequency"=w15:dbl, "VL Frequency"=w16:dbl, "Recloser action"=w216:bool, "Recloser out"=w150:cluster{bool, dbl})
    n169 = feedback-in #12(w150) -> ()
    n170 = call "Reclose.vi"("Recloser Settings"="Recloser Settings", "Recloser in"=w138, "Reclose?"="Reclose Relay4?", "VR RMS avg"=w134, "VL RMS avg"=w135, "VR array"=w137, "VL array"=w136) -> ("Phase difference"=w172:dbl, "VR Frequency"=w143:dbl, "VL Frequency"=w142:dbl, "Recloser action"=w215:bool, "Recloser out"=w139:cluster{bool, dbl})
    n171 = feedback-in #10(w139) -> ()
    n172 = call "Reclose.vi"("Recloser Settings"="Recloser Settings", "Recloser in"=w116, "Reclose?"="Reclose Relay6?", "VR RMS avg"=w114, "VL RMS avg"=w115, "VR array"=w118, "VL array"=w119) -> ("Phase difference"=w253:dbl, "VR Frequency"=w112:dbl, "VL Frequency"=w113:dbl, "Recloser action"=w213:bool, "Recloser out"=w117:cluster{bool, dbl})
    n173 = feedback-in #13(w117) -> ()
    n174 = feedback #14() -> (w98:cluster{bool, dbl})  [unwired: 1 in]
    n175 = call "Reclose.vi"("Recloser Settings"="Recloser Settings", "Recloser in"=w98, "Reclose?"="Reclose Relay8?", "VR RMS avg"=w96, "VL RMS avg"=w97, "VR array"=w101, "VL array"=w102) -> ("Phase difference"=w240:dbl, "VR Frequency"=w95:dbl, "VL Frequency"=w94:dbl, "Recloser action"=w211:bool, "Recloser out"=w99:cluster{bool, dbl})
    n176 = feedback-in #14(w99) -> ()
    n177 = feedback #15() -> (w167:cluster{bool, dbl})  [unwired: 1 in]
    n178 = call "Reclose.vi"("Recloser Settings"="Recloser Settings", "Recloser in"=w167, "Reclose?"="Reclose Relay1?", "VR RMS avg"=w163, "VL RMS avg"=w164, "VR array"=w165, "VL array"=w166) -> ("Phase difference"=w18:dbl, "VR Frequency"=w161:dbl, "VL Frequency"=w162:dbl, "Recloser action"=w289:bool, "Recloser out"=w168:cluster{bool, dbl})
    "Waveform Chart 2" <- w18
    n179 = feedback-in #15(w168) -> ()
    n180 = feedback #16() -> (w83:cluster{bool, dbl})  [unwired: 1 in]
    n181 = call "Reclose.vi"("Recloser Settings"="Recloser Settings", "Recloser in"=w83, "Reclose?"="Reclose Relay7?", "VR RMS avg"=w106, "VL RMS avg"=w107, "VR array"=w109, "VL array"=w110) -> ("Phase difference"=w279:dbl, "VR Frequency"=w104:dbl, "VL Frequency"=w105:dbl, "Recloser action"=w212:bool, "Recloser out"=w249:cluster{bool, dbl})
    n182 = feedback-in #16(w249) -> ()
    n183 = feedback #17() -> (w132:cluster{bool, dbl})  [unwired: 1 in]
    n184 = call "Reclose.vi"("Recloser Settings"="Recloser Settings", "Recloser in"=w132, "Reclose?"="Reclose Relay5?", "VR RMS avg"=w57, "VL RMS avg"=w128, "VR array"=w130, "VL array"=w131) -> ("Phase difference"=w259:dbl, "VR Frequency"=w125:dbl, "VL Frequency"=w126:dbl, "Recloser action"=w214:bool, "Recloser out"=w133:cluster{bool, dbl})
    n185 = feedback-in #17(w133) -> ()
    n186 = Index Array(array=w103) -> (element #1=w241:dbl, element #2=w242:dbl)  [unwired: 2 in]
    n187 = Index Array(array=w185) -> (element #1=w236:dbl, element #2=w245:dbl)  [unwired: 2 in]
    n188 = Index Array(array=w186) -> (element #1=w254:dbl, element #2=w255:dbl)  [unwired: 2 in]
    n189 = Index Array(array=w201) -> (element #1=w258:dbl, element #2=w257:dbl)  [unwired: 2 in]
    n190 = Index Array(array=w140) -> (element #1=w266:dbl, element #2=w267:dbl)  [unwired: 2 in]
    n191 = case shown="False" "Manual Relay Control" {
      tunnel: w213 -> [w501 _]
      frame False {
        n192 = local write "Relay6"(w501) -> ()
      }
      frame True {
      }
    }
    n193 = case shown="False" "Manual Relay Control" {
      tunnel: w211 -> [w499 _]
      frame False {
        n194 = local write "Relay8"(w499) -> ()
      }
      frame True {
      }
    }
    n195 = Index Array(array=w155) -> (element #1=w174:dbl, element #2=w173:dbl)  [unwired: 2 in]
    n196 = case shown="False" "Manual Relay Control" {
      tunnel: w214 -> [w502 _]
      frame False {
        n197 = local write "Relay5"(w502) -> ()
      }
      frame True {
      }
    }
    n198 = case shown="False" "Manual Relay Control" {
      tunnel: w212 -> [w500 _]
      frame False {
        n199 = local write "Relay7"(w500) -> ()
      }
      frame True {
      }
    }
    n200 = case shown="False" "Manual Relay Control" {
      tunnel: w289 -> [w562 _]
      frame False {
        n201 = local write "Relay1"(w562) -> ()
      }
      frame True {
      }
    }
    n202 = Index Array(array=w156) -> (element #1=w309:dbl, element #2=w394:dbl)  [unwired: 2 in]
    n203 = case shown="False" "Manual Relay Control" {
      tunnel: w216 -> [w504 _]
      frame False {
        n204 = local write "Relay3"(w504) -> ()
      }
      frame True {
      }
    }
    n205 = Index Array(array=w199) -> (element #1=w263:dbl, element #2=w270:dbl)  [unwired: 2 in]
    n206 = case shown="False" "Manual Relay Control" {
      tunnel: w215 -> [w503 _]
      frame False {
        n207 = local write "Relay4"(w503) -> ()
      }
      frame True {
      }
    }
    n208 = case shown="False" "Manual Relay Control" {
      tunnel: w217 -> [w505 _]
      frame False {
        n209 = local write "Relay2"(w505) -> ()
      }
      frame True {
      }
    }
    n210 = Index Array(array=w54) -> (element #2=w19:bool)  [unwired: 2 in, 1 out]
    n211 = Index Array(array=w53) -> (element #1=w30:bool, element #2=w33:bool)  [unwired: 2 in]
    n212 = Index Array(array=w52) -> (element #2=w42:bool)  [unwired: 2 in, 1 out]
    n213 = Index Array(array=w51) -> (element #1=w43:bool, element #2=w32:bool)  [unwired: 2 in]
    n214 = Index Array(array=w50) -> (element #1=w29:bool, element #2=w46:bool)  [unwired: 2 in]
    n215 = Index Array(array=w49) -> (element #1=w27:bool, element #2=w45:bool)  [unwired: 2 in]
    n216 = Index Array(array=w48) -> (element #1=w28:bool, element #2=w44:bool)  [unwired: 2 in]
    n217 = Index Array(array=w47) -> (element #1=w31:bool)  [unwired: 2 in, 1 out]
    n218 = Subtract(x=w151, y=w152) -> (x-y=w234:dbl)
    n219 = Subtract(x=w161, y=w162) -> (x-y=w312:dbl)
    n220 = local read "Relay8"() -> (w238:bool)
    n221 = local read "Relay5"() -> (w261:bool)
    n222 = local read "Relay3"() -> (w272:bool)
    n223 = local read "Relay6"() -> (w251:bool)
    n224 = local read "Relay7"() -> (w247:bool)
    n225 = local read "Relay2"() -> (w276:bool)
    n226 = local read "Relay4"() -> (w265:bool)
    n227 = local read "Relay1"() -> (w396:bool)
    n228 = Unbundle By Name(w284) -> ("Direction"=w200:enum16{"forward", "backward", "N/D"})
    n229 = Boolean To (0,1)(Boolean=w238) -> (0, 1=w239:i16)
    n230 = Build Array(w239, w97, w96, w94, w95, w240, w241, w242, w243, w243) -> (w324:dbl[])
    "R8 Data for\ncommunication" <- w324
    n231 = Boolean To (0,1)(Boolean=w261) -> (0, 1=w260:i16)
    n232 = Build Array(w260, w128, w57, w126, w125, w259, w258, w257, w127, w127) -> (w327:dbl[])
    "R5 Data for\ncommunication" <- w327
    n233 = Unbundle By Name(w55) -> ("Direction"=w191:enum16{"forward", "backward", "N/D"})
    n234 = Boolean To (0,1)(Boolean=w272) -> (0, 1=w271:i16)
    n235 = Build Array(w271, w148, w147, w16, w15, w17, w263, w270, w269, w269) -> (w329:dbl[])
    "R3 Data for\ncommunication" <- w329
    n236 = Boolean To (0,1)(Boolean=w251) -> (0, 1=w252:i16)
    n237 = Build Array(w252, w115, w114, w113, w112, w253, w254, w255, w256, w256) -> (w326:dbl[])
    "R6 Data for\ncommunication" <- w326
    n238 = Boolean To (0,1)(Boolean=w247) -> (0, 1=w246:i16)
    n239 = Build Array(w246, w107, w106, w105, w104, w279, w236, w245, w244, w244) -> (w325:dbl[])
    "R7 Data for\ncommunication" <- w325
    n240 = Boolean To (0,1)(Boolean=w276) -> (0, 1=w277:i16)
    n241 = Build Array(w277, w153, w58, w152, w151, w171, w174, w173, 0.0 ("element"), w234) -> (w330:dbl[])
    "R2 Data for\ncommunication" <- w330
    n242 = Boolean To (0,1)(Boolean=w265) -> (0, 1=w141:i16)
    n243 = Build Array(w141, w135, w134, w142, w143, w172, w266, w267, w268, w268) -> (w328:dbl[])
    "R4 Data for\ncommunication" <- w328
    n244 = Unbundle By Name(w194) -> ("Direction"=w193:enum16{"forward", "backward", "N/D"})
    n245 = Unbundle By Name(w189) -> ("Direction"=w188:enum16{"forward", "backward", "N/D"})
    n246 = Boolean To (0,1)(Boolean=w396) -> (0, 1=w395:i16)
    n247 = Build Array(w395, w164, w163, w162, w161, w18, w309, w394, 0.0 ("element"), w312) -> (w331:dbl[])
    "R1 Data for\ncommunication" <- w331
    n248 = Unbundle By Name(w56) -> ("Direction"=w198:enum16{"forward", "backward", "N/D"})
    n249 = Unbundle By Name(w196) -> ("Direction"=w197:enum16{"forward", "backward", "N/D"})
    n250 = Compound Arithmetic op=OR(w42, w30, w43, w29, w27, w28, w31) -> (w41:bool)
    n251 = Compound Arithmetic op=OR(w19, w43, w27, w31, w29, w28) -> (w40:bool)
    n252 = Compound Arithmetic op=OR(w19, w30, w29, w43, w27, w28, w31) -> (w39:bool)
    n253 = Compound Arithmetic op=OR(w19, w33, w27, w42, w31, w29, w28) -> (w38:bool)
    n254 = Compound Arithmetic op=OR(w30, w19, w33, w32, w28, w27, w31, w19) -> (w37:bool)
    n255 = Compound Arithmetic op=OR(w33, w32, w46, w28, w31, w33) -> (w36:bool)
    n256 = Compound Arithmetic op=OR(w32, w46, w45, w31, w33, w19) -> (w35:bool)
    n257 = Compound Arithmetic op=OR(w46, w45, w44, w33, w32) -> (w34:bool)
    n258 = case shown="\"backward\"" w200 {
      tunnel: w283 -> [w497 _]
      frame "forward", Default {
        "R2 Transfer" <- w497
      }
      frame "backward" {
        n259 = local write "R2 Transfer"(FALSE ("R2 Transfer")) -> ()
      }
    }
    n260 = case shown="\"backward\"" w191 {
      tunnel: w190 -> [w489 _]
      frame "forward", Default {
        "R7 Transfer" <- w489
      }
      frame "backward" {
        n261 = local write "R7 Transfer"(FALSE ("R2 Transfer")) -> ()
      }
    }
    n262 = local write "R2 Blocking in"(w40) -> ()
    n263 = local write "R3 Blocking in"(w39) -> ()
    n264 = local write "R4 Blocking in"(w38) -> ()
    n265 = local write "R5 Blocking in"(w37) -> ()
    n266 = local write "R6 Blocking in"(w36) -> ()
    n267 = local write "R7 Blocking in"(w35) -> ()
    n268 = local write "R8 Blocking in"(w34) -> ()
    n269 = local write "R1 Blocking in"(w41) -> ()
    n270 = Subtract(x=w105, y=w104) -> (x-y=w278:dbl)
    n271 = case shown="\"forward\", Default" w193 {
      tunnel: w192 -> [w491 _]
      frame "forward", Default {
        "R5 Transfer" <- w491
      }
      frame "backward" {
        n272 = local write "R5 Transfer"(FALSE ("R2 Transfer")) -> ()
      }
    }
    n273 = case shown="\"forward\", Default" w188 {
      tunnel: w187 -> [w487 _]
      frame "forward", Default {
        "R8 Transfer" <- w487
      }
      frame "backward" {
        n274 = local write "R8 Transfer"(FALSE ("R2 Transfer")) -> ()
      }
    }
    n275 = shared-variable "IntelliRupter\\IntelliRupter_data.lvlib\\Relay7_Ang_Diff"(w279) -> ()  [unwired: 1 in, 1 out]
    n276 = case shown="\"forward\", Default" w197 {
      tunnel: w195 -> [w493 _]
      tunnel: [w493 FALSE] -> w281
      frame "forward", Default {
      }
      frame "backward" {
      }
    }
    n277 = shared-variable "IntelliRupter\\IntelliRupter_data.lvlib\\Relay7_Freq_Diff"(w278) -> ()  [unwired: 1 in, 1 out]
    n278 = case shown="\"forward\", Default" w198 {
      tunnel: w59 -> [w495 _]
      tunnel: [w495 FALSE] -> w282
      frame "forward", Default {
      }
      frame "backward" {
      }
    }
    n279 = Build Array (concatenate)(w331, w330, w329, w328, w327, w326, w325, w324) -> (w332:dbl[])
    n280 = Or(x=w282, y=w281) -> (x .or. y?=→"R4 Transfer":bool)
    n281 = shared-variable "IntelliRupter\\IntelliRupter_data.lvlib\\Relay_to_MGCC"(w332) -> ()  [unwired: 1 in, 1 out]
    n282 = shared-variable "IntelliRupter\\IntelliRupter_data.lvlib\\Relay7_Cmd"("Relay7") -> ()  [unwired: 1 in, 1 out]
    n283 = xnode "Read/Write Control"("FPGA VI Reference In"=w407, "Relay1"="Relay1", "Relay2"="Relay2", "Relay3"="Relay3", "Relay4"="Relay4", "Relay5"="Relay5", "Relay6"="Relay6", "Relay7"="Relay7", "Relay8"="Relay8", "Count(ticks)"="Count(ticks)") -> ("FPGA VI Reference Out"=w409:refnum<k20>, "error out"=w408:errorcluster)  [unwired: 1 in]
    n284 = node-c288() -> ()  [unwired: 1 in, 1 out]
  }
  n285 = node-c288(w3) -> ()  [unwired: 1 out]
  n286 = xnode "Close FPGA VI Reference"("FPGA VI Reference In"=w13, "error in"=w12) -> ()  [unwired: 1 out]
